vi "ClawController.vi"(10 "SensorInputData":T1, 11 "HMI to Control":T2) -> (2 "Claw Intake Value":dbl, 3 "Claw Final Output":dbl)   [LabVIEW 2014]
uses:
  Typedefs/HMI_to_Control.ctl
  Typedefs/Arm States.ctl
  Typedefs/ClawStates.ctl
  Typedefs/IntakeWheelSenseOrManual.ctl
  Typedefs/SensorInputData.ctl
  Gensubs/Bert_or_Ernie.vi
panel:
  out "Setpoint vs. PV.":cluster{"ClawWidth":dbl, "Setpoint":dbl}(graph)
  # "Mike Look Here!"
  # "Value must remain\nbetween 0 and 1\n\nif not get Jim!"
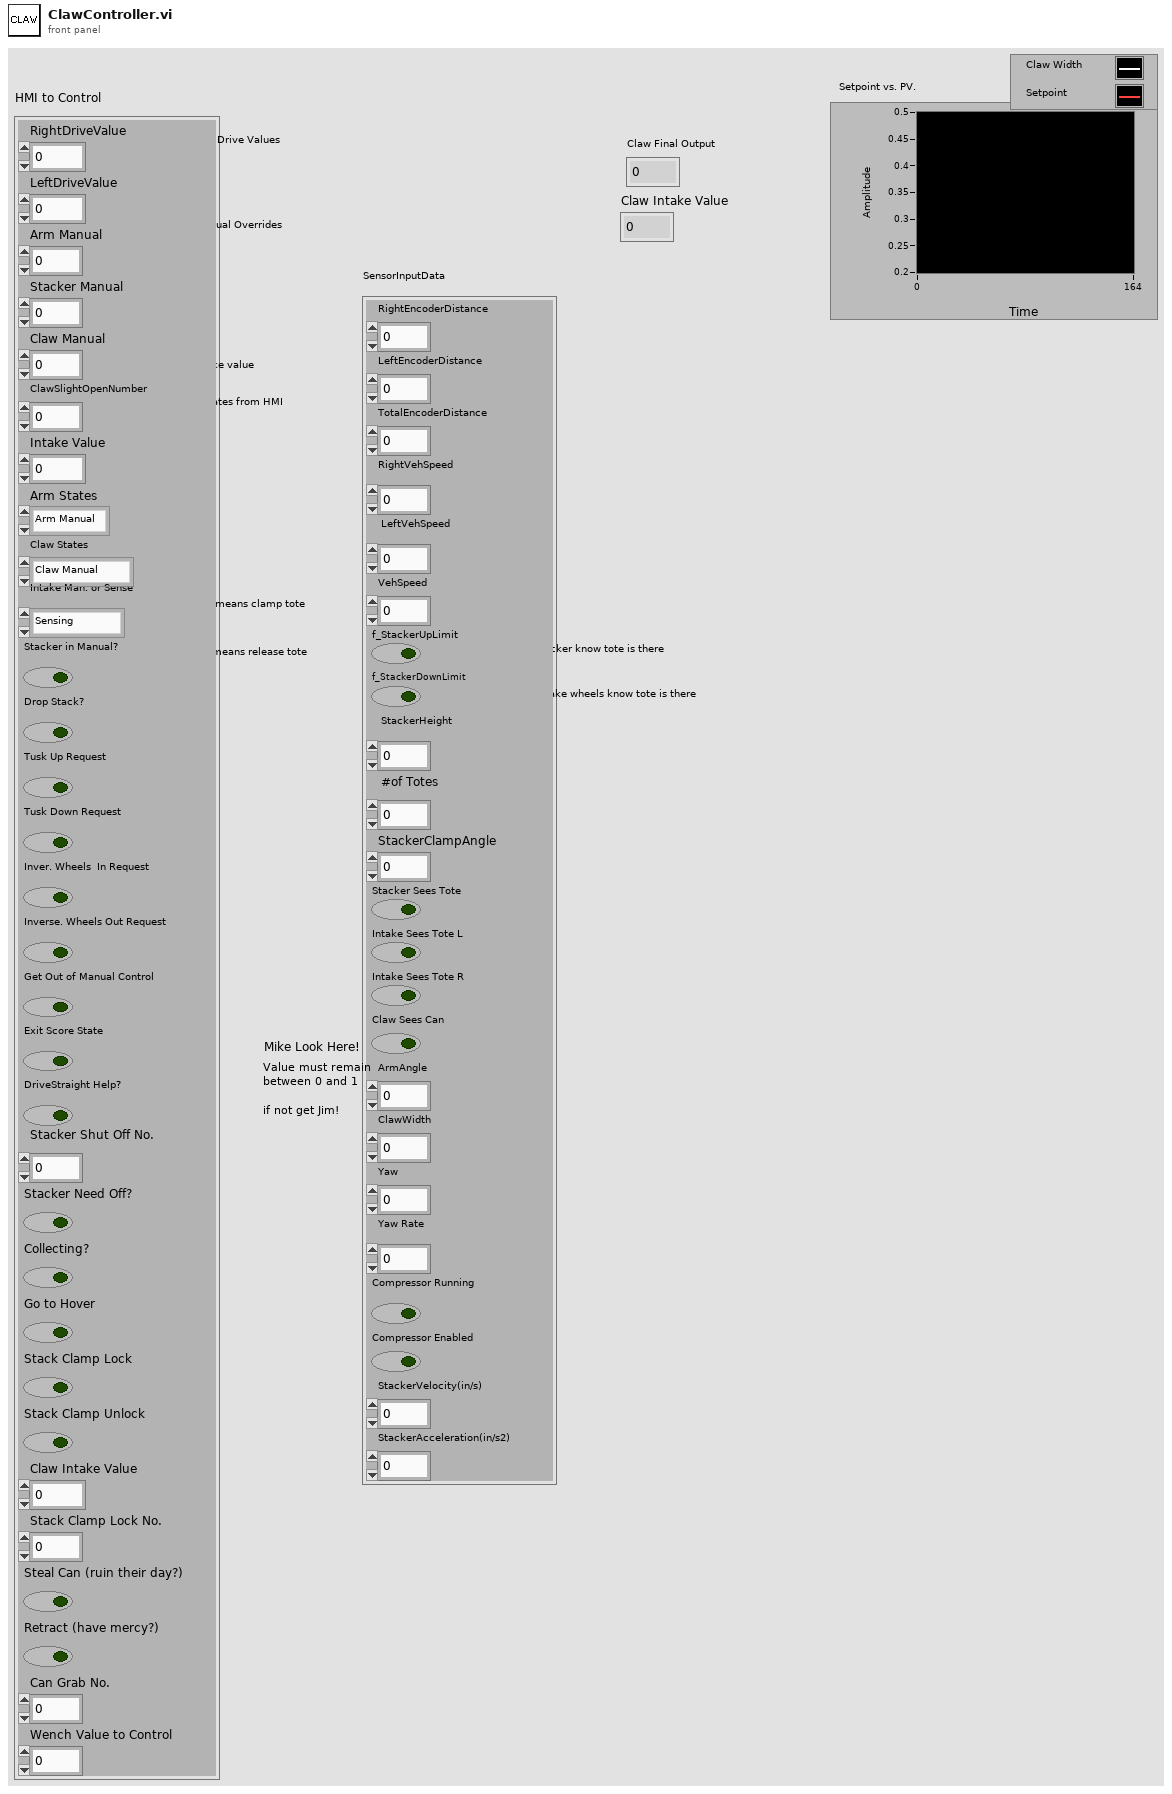
[diagram p1: front panel]
types:
  T1 = typedef "SensorInputData.ctl" = cluster{"RightEncoderDistance":dbl, "LeftEncoderDistance":dbl, "TotalEncoderDistance":dbl, "RightVehSpeed":dbl, "LeftVehSpeed":dbl, "VehSpeed":dbl, "f_StackerUpLimit":bool, "f_StackerDownLimit":bool, "StackerHeight":dbl, "#of Totes":u8, "StackerClampAngle":dbl, "Stacker Sees Tote":bool, "Intake Sees Tote L":bool, "Intake Sees Tote R":bool, "Claw Sees Can":bool, "ArmAngle":dbl, "ClawWidth":dbl, "Yaw":dbl, "Yaw Rate":dbl, "Compressor Running":bool, "Compressor Enabled":bool, "StackerVelocity(in/s)":dbl, "StackerAcceleration(in/s2)":dbl}
  T2 = typedef "HMI_to_Control.ctl" = cluster{"RightDriveValue":dbl, "LeftDriveValue":dbl, "Arm Manual ":dbl, "Stacker Manual ":dbl, "Claw Manual ":dbl, "ClawSlightOpenNumber":i8, "Intake Value ":sgl, "Arm States":T3, "Claw States":T4, "Intake Man. or Sense":T5, "Stacker in Manual?":bool, "Drop Stack? ":bool, "Tusk Up Request":bool, "Tusk Down Request":bool, "Inver. Wheels  In Request":bool, "Inverse. Wheels Out Request ":bool, "Get Out of Manual Control":bool, "Exit Score State":bool, "DriveStraight Help?":bool, "Stacker Shut Off No.":i8, "Stacker Need Off?":bool, "Collecting?":bool, "Go to Hover":bool, "Stack Clamp Lock ":bool, "Stack Clamp Unlock ":bool, "Claw Intake Value ":sgl, "Stack Clamp Lock No. ":i8, "Steal Can (ruin their day?)":bool, "Retract (have mercy?)":bool, "Can Grab No. ":i8, "Wench Value to Control ":dbl}
  T3 = typedef "Arm States.ctl" = enum16{"Arm Manual ", "Ground", "Step", "1 Tote", "2 Tote", "3 Tote", "4 Tote", "5 Tote", "6 Tote", "Flip Can Arm", "Grab Can in auto", "Nudge"}
  T4 = typedef "ClawStates.ctl" = enum16{"Claw Manual ", "Claw Open", "Claw Closed", "Claw Slight Open", "Flip Can"}
  T5 = typedef "IntakeWheelSenseOrManual.ctl" = enum16{"Sensing", "Manual "}
  T6 = cluster{"Arm_kP":dbl, "Arm_kI":dbl, "Arm_kD":dbl}
  T7 = enum16{"Slight Please", "Now Flip Can", "Check Slight"}
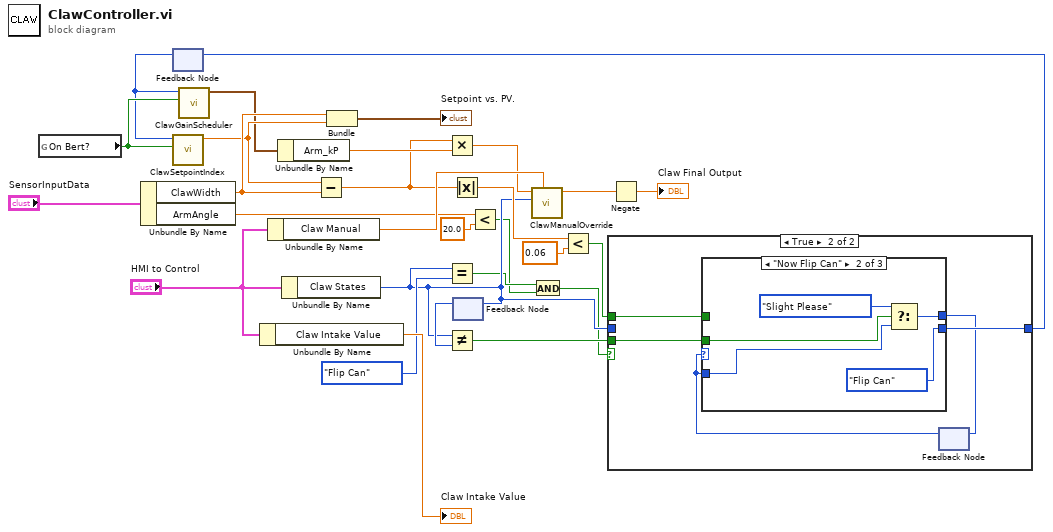
[diagram p0: block diagram]
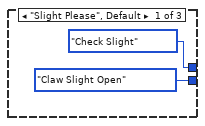
[diagram p3: hidden frame]
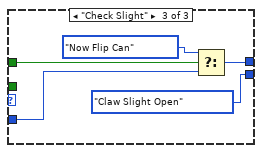
[diagram p4: hidden frame]
diagram:
  n1 = global read "Bert_or_Ernie.vi" "On Bert?"() -> (w18:bool)
  n2 = Unbundle By Name("SensorInputData") -> ("ClawWidth"=w27:dbl, "ArmAngle"=w3:dbl)
  n3 = feedback #1() -> (w9:T4)  [unwired: 1 in]
  n4 = call "ClawSetpointIndex.vi"("On Bert?"=w18, "Claw States"=w9) -> ("Setpoint"=w26:dbl)  [unwired: 9 in]
  n5 = call "ClawGainScheduler.vi"("On Bert?"=w18, "Claw States"=w9) -> ("ClawGainsOut"=w22:T6)  [unwired: 9 in]
  n6 = Unbundle By Name("HMI to Control") -> ("Claw Intake Value"=→"Claw Intake Value":sgl)
  n7 = Unbundle By Name("HMI to Control") -> ("Claw Manual"=w24:dbl)
  n8 = Unbundle By Name(w22) -> ("Arm_kP"=w21:dbl)
  n9 = Unbundle By Name("HMI to Control") -> ("Claw States"=w7:T4)
  n10 = Subtract(x=w26, y=w27) -> (x-y=w14:dbl)
  n11 = Bundle("ClawWidth"=w27, "Setpoint"=w26) -> (→"Setpoint vs. PV.":cluster{"ClawWidth":dbl, "Setpoint":dbl})  [unwired: 1 in]
  n12 = Multiply(x=w14, y=w21) -> (x*y=w23:dbl)
  n13 = Equal?(x=w7, y=ClawStates."Flip Can") -> (x = y?=w5:bool)
  n14 = Absolute Value(x=w14) -> (abs(x)=w13:dbl)
  n15 = feedback-in #2(w7) -> ()
  n16 = feedback #2() -> (w8:T4)  [unwired: 1 in]
  n17 = Not Equal?(x=w7, y=w8) -> (x != y?=w6:bool)
  n18 = Less?(x=w3, y=20.0) -> (x < y?=w1:bool)
  n19 = call "ClawManualOverride.vi"("Claw Manual Input"=w24, "Claw States"=w7, "Claw PID Input"=w23) -> ("Claw Output"=w20:dbl)  [unwired: 8 in]
  n20 = And(x=w5, y=w1) -> (x .and. y?=w4:bool)
  n21 = Less?(x=w13, y=0.06) -> (x < y?=w11:bool)
  n22 = case shown="True" w4 {
    tunnel: w7 -> [w29 _]
    tunnel: [w29 w34] -> w10
    tunnel: w11 -> [_ w32]
    tunnel: w6 -> [_ w30]
    frame False {
    }
    frame True {
      n23 = feedback #3() -> (w31:T7)  [unwired: 1 in]
      n24 = case shown="\"Now Flip Can\"" w31 {
        tunnel: [ClawStates."Claw Slight Open" ("Claw States") ClawStates."Flip Can" ("Claw States") ClawStates."Claw Slight Open" ("Claw States")] -> w34
        tunnel: [T7."Check Slight" w37 w42] -> w33
        tunnel: w32 -> [_ _ w45]
        tunnel: w31 -> [_ w38 w43]
        tunnel: w30 -> [_ w40 _]
        frame "Slight Please", Default {
        }
        frame "Now Flip Can" {
          n25 = Select(t=T7."Slight Please", s=w40, f=w38) -> (s? t:f=w37:T7)
        }
        frame "Check Slight" {
          n26 = Select(t=T7."Now Flip Can", s=w45, f=w43) -> (s? t:f=w42:T7)
        }
      }
      n27 = feedback-in #3(w33) -> ()
    }
  }
  n28 = feedback-in #1(w10) -> ()
  n29 = Negate(x=w20) -> (-x=→"Claw Final Output":dbl)
